vi "Init.vi"(7 "Value Type":T1=enum."Object", 8 "error in (no error)":errorcluster, 9 "Meta Data":T2[](array[typedef]), 10 "Value":variant, 11 "Name":string) -> (0 "error out":errorcluster, 3 "Config Element out":refnum<class "Config Element.lvclass">)   [LabVIEW 2020, in "CDM-Config.lvlib" / "Config Element.lvclass"]
uses:
  Config Element.lvclass
  Meta Data.ctl
  Value Type.ctl
  Ref Data.ctl
  Node Info.ctl
  Config Element.lvclass/Config Element.ctl
  CDM-Config.lvlib
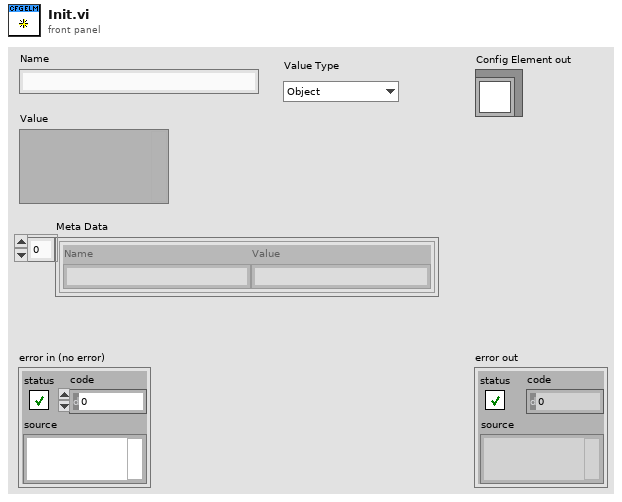
[diagram p1: front panel]
types:
  T1 = typedef "CDM-Config.lvlib/Value Type.ctl" = enum16{"String", "Number", "Bool", "Object", "Array"}
  T2 = typedef "CDM-Config.lvlib/Meta Data.ctl" = cluster{"Name":string, "Value":string}
  T3 = typedef "CDM-Config.lvlib/Config Element.lvclass/Ref Data.ctl" = cluster{"Node Info":T4, "Owner":refnum<class>, "Changed":bool, "Name":string, "Meta Data":T2[], "Value Type":T1, "Value":variant}
  T4 = typedef "CDM-Config.lvlib/Node Info.ctl" = cluster{"Index":i32, "Parent":i32, "Children":i32[]}
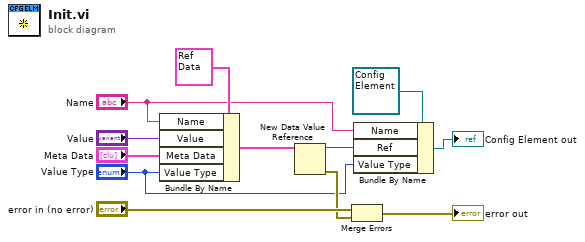
[diagram p0: block diagram]
diagram:
  n1 = Bundle By Name(cluster=T3 {"Node Info"={"Index"=0, "Parent"=0, "Children"=[]}, "Owner"=refnum, "Changed"=FALSE, "Name"="", "Meta Data"=[], "Value Type"=enum."String", "Value"=variant(string "")} ("Ref Data"), "Name"="Name", "Value"="Value", "Meta Data"="Meta Data", "Value Type"="Value Type") -> (w5:T3)
  n2 = New Data Value Reference(data value=w5) -> (data value reference=w8:refnum<data-value>, error out=w6:errorcluster)  [unwired: 1 in]
  n3 = Merge Errors("error in (no error)", w6) -> (→"error out":errorcluster)
  n4 = Bundle By Name(cluster=refnum<class "Config Element.lvclass"> refnum ("Config Element in"), "Name"="Name", "Ref"=w8, "Value Type"="Value Type") -> (→"Config Element out":refnum<class "Config Element.lvclass">)
